vi "getSecNameFromSecvarExp.vi"(11 "secvarExp":string) -> (3 "secWith*":string)   [LabVIEW 2010]
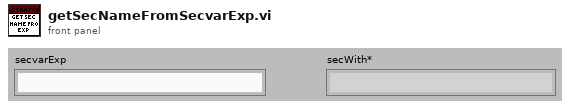
[diagram p1: front panel]
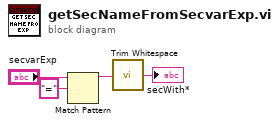
[diagram p0: block diagram]
diagram:
  n1 = Match Pattern(string="secvarExp", regular expression="=") -> (before substring=w3:string)  [unwired: 1 in, 3 out]
  n2 = call <vilib>:"Trim Whitespace.vi"("string"=w3) -> ("trimmed string"=→"secWith*":string)  [unwired: 1 in]
